vi "PZT voltage set.vi"(2 "error in (no error)":errorcluster caption="错误输入（无错误）", 3 "电压值（V）":i32, 4 "VISA resource name":refnum<visa-resource-name> caption="VISA资源名称") -> (0 "错误输出":errorcluster, 1 "VISA资源名称输出":refnum<visa-resource-name>)   [LabVIEW 2019]
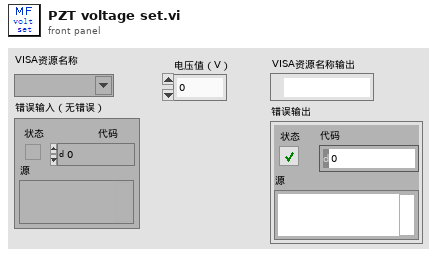
[diagram p1: front panel]
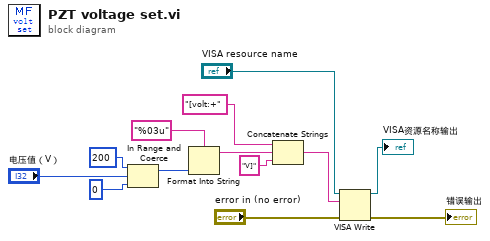
[diagram p0: block diagram]
diagram:
  n1 = In Range and Coerce(upper limit=200 ("上限"), x="电压值（V）", lower limit=0 ("下限")) -> (coerced(x)=w3:i32)  [unwired: 1 out]
  n2 = Format Into String(format string="%03u" ("格式字符串"), w3) -> (resulting string=w9:string)  [unwired: 2 in, 1 out]
  n3 = Concatenate Strings("[volt:+" ("字符串"), w9, "V]" ("字符串")) -> (w6:string)
  n4 = VISA Write(VISA resource name="VISA resource name", write buffer=w6, error in (no error)="error in (no error)") -> (VISA resource name out=→"VISA资源名称输出":refnum<visa-resource-name>, error out=→"错误输出":errorcluster)  [unwired: 1 out]
